vi "Robo Team Update GUI Control by Status.vi"(11 "Status":T1) -> ()   [LabVIEW 2015]
uses:
  RT Controls/LP Status typedef.ctl
  Robo Team Globals.vi
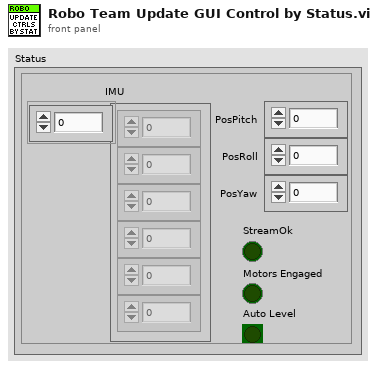
[diagram p1: front panel]
types:
  T1 = typedef "LP Status typedef.ctl" = cluster{"PosPitch":dbl, "PosRoll":dbl, "PosYaw":dbl, "IMU":dbl[], "StreamOk":bool, "Motors Engaged":bool, "Auto Level":bool}
  T2 = typedef "Robo Axis Ref.ctl" = cluster{"Pitch Angle":refnum<vi>, "Roll Angle":refnum<vi>, "Yaw Angle":refnum<vi>, "Pitch IMU":refnum<vi>, "Roll IMU":refnum<vi>, "Yaw IMU":refnum<vi>, "Pitch Angle Digit":refnum<vi>, "Roll Angle Digit":refnum<vi>, "Yaw Angle Digit":refnum<vi>}
  T3 = enum8{"Enabled", "Disabled", "Disabled and Grayed Out"}
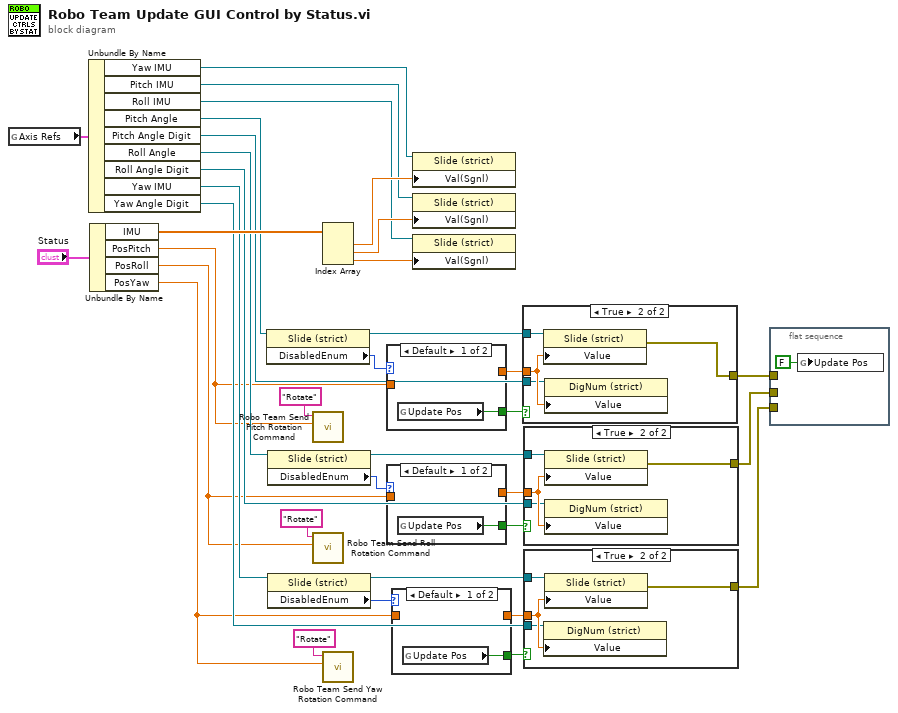
[diagram p0: block diagram]
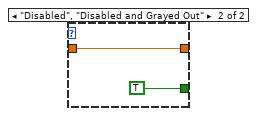
[diagram p2: hidden frame]
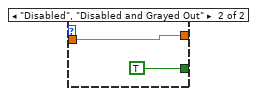
[diagram p3: hidden frame]
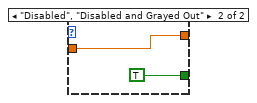
[diagram p4: hidden frame]
diagram:
  n1 = global read "Robo Team Globals.vi" "Axis Refs"() -> (w29:T2)
  n2 = Unbundle By Name(w29) -> ("Yaw IMU"=w30:refnum<vi>, "Pitch IMU"=w31:refnum<vi>, "Roll IMU"=w32:refnum<vi>, "Pitch Angle"=w27:refnum<vi>, "Pitch Angle Digit"=w21:refnum<vi>, "Roll Angle"=w24:refnum<vi>, "Roll Angle Digit"=w20:refnum<vi>, "Yaw IMU"=w22:refnum<vi>, "Yaw Angle Digit"=w19:refnum<vi>)
  n3 = Unbundle By Name("Status") -> ("IMU"=w33:dbl[], "PosPitch"=w6:dbl, "PosRoll"=w4:dbl, "PosYaw"=w2:dbl)
  n4 = property class="Slide (strict)"(reference=w27) -> (reference out=w26:refnum<vi>, "DisabledEnum"=w18:T3)  [unwired: 1 in, 1 out]
  n5 = property class="Slide (strict)"(reference=w24) -> (reference out=w25:refnum<vi>, "DisabledEnum"=w16:T3)  [unwired: 1 in, 1 out]
  n6 = property class="Slide (strict)"(reference=w22) -> (reference out=w23:refnum<vi>, "DisabledEnum"=w14:T3)  [unwired: 1 in, 1 out]
  n7 = call "Robo Team Send Pitch Rotation Command.vi"("Data in"=w6, "Command"="Rotate") -> ()  [unwired: 8 in, 2 out]
  n8 = call "Robo Team Send Roll Rotation Command.vi"("Data in"=w4, "Command"="Rotate") -> ()  [unwired: 8 in, 2 out]
  n9 = Index Array(array=w33) -> (element #1=w34:dbl, element #2=w35:dbl, element #3=w36:dbl)  [unwired: 3 in]
  n10 = call "Robo Team Send Yaw Rotation Command.vi"("Data in"=w2, "Command"="Rotate") -> ()  [unwired: 8 in, 2 out]
  n11 = case shown="Default" w18 {
    tunnel: [w37 TRUE] -> w17
    tunnel: w6 -> [_ w38]
    tunnel: [_ w38] -> w5
    frame Default {
      n12 = global read "Robo Team Globals.vi" "Update Pos"() -> (w37:bool)
    }
    frame "Disabled", "Disabled and Grayed Out" {
    }
  }
  n13 = case shown="Default" w16 {
    tunnel: [w40 TRUE] -> w15
    tunnel: w4 -> [_ w41]
    tunnel: [_ w41] -> w3
    frame Default {
      n14 = global read "Robo Team Globals.vi" "Update Pos"() -> (w40:bool)
    }
    frame "Disabled", "Disabled and Grayed Out" {
    }
  }
  n15 = case shown="Default" w14 {
    tunnel: [w43 TRUE] -> w13
    tunnel: [_ w44] -> w1
    tunnel: w2 -> [_ w44]
    frame Default {
      n16 = global read "Robo Team Globals.vi" "Update Pos"() -> (w43:bool)
    }
    frame "Disabled", "Disabled and Grayed Out" {
    }
  }
  n17 = property class="Slide (strict)"(reference=w30, "Val(Sgnl)"=w34) -> ()  [unwired: 1 in, 2 out]
  n18 = property class="Slide (strict)"(reference=w31, "Val(Sgnl)"=w35) -> ()  [unwired: 1 in, 2 out]
  n19 = property class="Slide (strict)"(reference=w32, "Val(Sgnl)"=w36) -> ()  [unwired: 1 in, 2 out]
  n20 = case shown="True" w17 {
    tunnel: w26 -> [_ w49]
    tunnel: w5 -> [_ w48]
    tunnel: w21 -> [_ w47]
    tunnel: [_ w46] -> w12
    frame False {
    }
    frame True {
      n21 = property class="Slide (strict)"(reference=w49, "Value"=w48) -> (error out=w46:errorcluster)  [unwired: 1 in, 1 out]
      n22 = property class="DigNum (strict)"(reference=w47, "Value"=w48) -> ()  [unwired: 1 in, 2 out]
    }
  }
  n23 = case shown="True" w15 {
    tunnel: w25 -> [_ w53]
    tunnel: w3 -> [_ w52]
    tunnel: w20 -> [_ w51]
    tunnel: [_ w50] -> w11
    frame False {
    }
    frame True {
      n24 = property class="Slide (strict)"(reference=w53, "Value"=w52) -> (error out=w50:errorcluster)  [unwired: 1 in, 1 out]
      n25 = property class="DigNum (strict)"(reference=w51, "Value"=w52) -> ()  [unwired: 1 in, 2 out]
    }
  }
  n26 = case shown="True" w13 {
    tunnel: w23 -> [_ w57]
    tunnel: w1 -> [_ w56]
    tunnel: w19 -> [_ w55]
    tunnel: [_ w54] -> w10
    frame False {
    }
    frame True {
      n27 = property class="DigNum (strict)"(reference=w55, "Value"=w56) -> ()  [unwired: 1 in, 2 out]
      n28 = property class="Slide (strict)"(reference=w57, "Value"=w56) -> (error out=w54:errorcluster)  [unwired: 1 in, 1 out]
    }
  }
  n29 = flat-sequence {
    tunnel: w12 -> [_]
    tunnel: w11 -> [_]
    tunnel: w10 -> [_]
    frame #0 {
      n30 = global write "Robo Team Globals.vi" "Update Pos"(FALSE ("Update Pos")) -> ()
    }
  }
